vi "Lockin.Low Pass Filter (subVI).vi"(6 "Butterworth? [T]":bool=TRUE, 8 "error in (no error)":errorcluster, 9 "Element Data":i32, 10 "signal in":waveform(dbl)[](array[waveform]), 11 "DSP in":refnum<class "DSP.lvclass">) -> (0 "error out":errorcluster, 1 "Fc (Hz)":dbl, 2 "signal out":waveform(dbl)[](array[waveform]), 3 "DSP out":refnum<class "DSP.lvclass">)   [LabVIEW 2019, in "DSP.lvclass"]
uses:
  DSP.lvclass
  DSP.lvclass/DSP.ctl
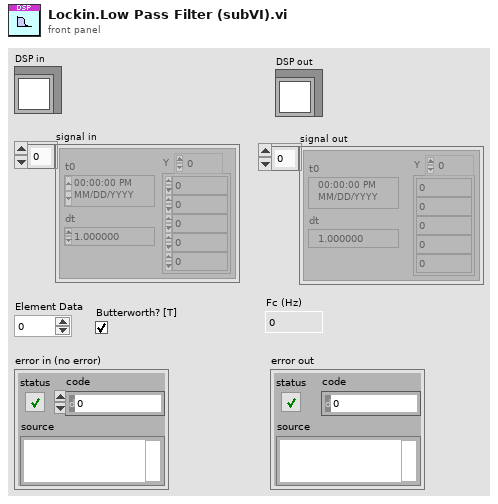
[diagram p1: front panel]
types:
  T1 = typedef "DSP.lvclass/REF.Channel--Cluster--Array.ctl" = T2[]
  T2 = typedef "DSP.lvclass/REF.Channel--Cluster.ctl" = cluster{"Enable?":bool, "Channel":i32, "Frequency":dbl, "Phase":dbl, "TC":dbl, "Roll-Off":i32}
  T3 = cluster{"filter structure":enum32{"IIR 2nd Order", "IIR 4th Order"}, "Reverse Coefficients":dbl[], "Forward Coefficients":dbl[]}[]
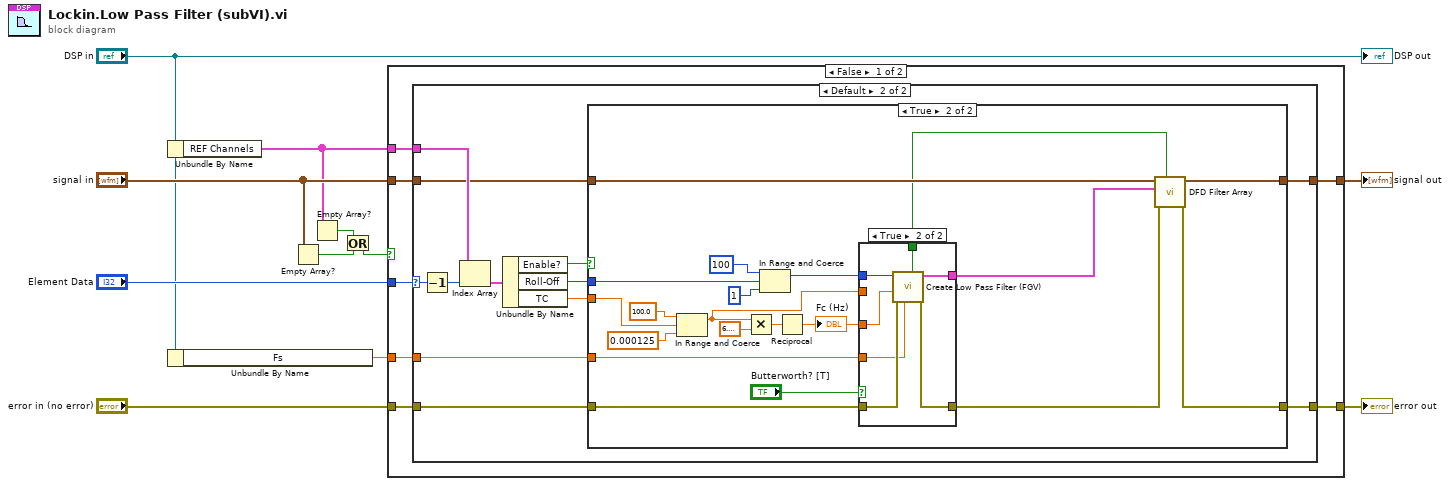
[diagram p0: block diagram]
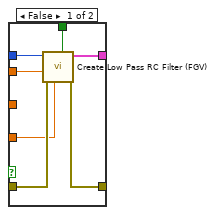
[diagram p4: hidden frame]
diagram:
  n1 = Unbundle By Name("DSP in") -> ("REF Channels"=w6:T1)
  n2 = Unbundle By Name("DSP in") -> ("Fs"=w1:dbl)
  n3 = Empty Array?(array="signal in") -> (empty?=w4:bool)
  n4 = Empty Array?(array=w6) -> (empty?=w5:bool)
  n5 = Or(x=w5, y=w4) -> (x .or. y?=w3:bool)
  n6 = case shown="False" w3 {
    tunnel: "error in (no error)" -> [w18 w70]
    tunnel: [w17 w70] -> w10
    tunnel: [w16 w69] -> w9
    tunnel: "Element Data" -> [w14 _]
    tunnel: "signal in" -> [w15 w69]
    tunnel: w6 -> [w13 _]
    tunnel: w1 -> [w12 _]
    frame False {
      n7 = case shown="Default" w14 {
        selector: w14 -> [_ w30]
        tunnel: w18 -> [w20 w24]
        tunnel: [w20 w25] -> w17
        tunnel: w15 -> [w19 w27]
        tunnel: [w19 w26] -> w16
        tunnel: w13 -> [_ w28]
        tunnel: w12 -> [_ w22]
        frame 0 {
        }
        frame Default {
          n8 = Decrement(x=w30) -> (x-1=w29:i32)
          n9 = Index Array(array=w28, index=w29) -> (element=w32:T2)
          n10 = Unbundle By Name(w32) -> ("Enable?"=w21:bool, "Roll-Off"=w23:i32, "TC"=w31:dbl)
          n11 = case shown="True" w21 {
            tunnel: w31 -> [_ w54]
            tunnel: w27 -> [w34 w47]
            tunnel: [w34 w46] -> w26
            tunnel: [w33 w45] -> w25
            tunnel: w24 -> [w33 w44]
            tunnel: w23 -> [_ w40]
            tunnel: w22 -> [_ w39]
            frame False {
            }
            frame True {
              n12 = In Range and Coerce(upper limit=100.0, x=w54, lower limit=0.000125) -> (coerced(x)=w35:dbl)  [unwired: 1 out]
              n13 = Multiply(x=w35, y=6.283185307179586) -> (x*y=w51:dbl)
              n14 = In Range and Coerce(upper limit=100, x=w40, lower limit=1) -> (coerced(x)=w43:i32)  [unwired: 1 out]
              n15 = Reciprocal(x=w51) -> (1/x=w38:dbl)
              "Fc (Hz)" <- w38
              n16 = case shown="True" "Butterworth? [T]" {
                tunnel: w44 -> [w57 w68]
                tunnel: w43 -> [w61 w67]
                tunnel: [w58 w66] -> w42
                tunnel: [w59 w65] -> w36
                tunnel: [w60 w64] -> w41
                tunnel: w39 -> [w55 w63]
                tunnel: w38 -> [_ w62]
                tunnel: w35 -> [w56 _]
                frame False {
                  n17 = call "Create Low Pass RC Filter (FGV).vi"("fs (Hz)"=w55, "error in (no error)"=w57, "time constant (s)"=w56, "stages"=w61) -> ("error out"=w58:errorcluster, "IIR Filters"=w60:T3, "init out"=w59:bool)  [unwired: 5 in]
                }
                frame True {
                  n18 = call "Create Low Pass Filter (FGV).vi"("fs (Hz)"=w63, "error in (no error)"=w68, "Low Pass Cutoff (Hz)"=w62, "order"=w67) -> ("error out"=w66:errorcluster, "IIR Filters"=w64:T3, "init out"=w65:bool)  [unwired: 5 in]
                }
              }
              n19 = call "DFD Filter Array.vi"("init (F)"=w36, "error in (no error)"=w42, "IIR Filters"=w41, "signal in"=w47) -> ("error out"=w45:errorcluster, "signal out"=w46:waveform(dbl)[])  [unwired: 6 in]
            }
          }
        }
      }
    }
    frame True {
    }
  }
  "error out" <- w10
  "signal out" <- w9
  "DSP out" <- "DSP in"
